vi "precess_SN.vi"() -> ()   [LabVIEW 2010]
panel:
  out "STR":dbl format="%.12g"
  out "DEC 2":dbl caption="DEC 2 [°.xxxxxx]" format="%.6g"
  out "RA 2":dbl caption="RA 2 [h.xxxxxx]" format="%.6g"
  in  "EPOCH2":dbl caption="EPOCH 2" format="%.3g"
  in  "EPOCH1":dbl caption="EPOCH 1" format="%.3g"
  in  "DEC 1":dbl caption="DEC 1 [°.xxxxxx]" format="%.6g"
  in  "RA 1":dbl caption="RA 1 [h.xxxxxx]" format="%.6g"
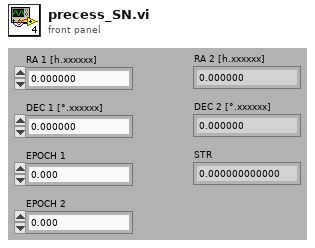
[diagram p1: front panel]
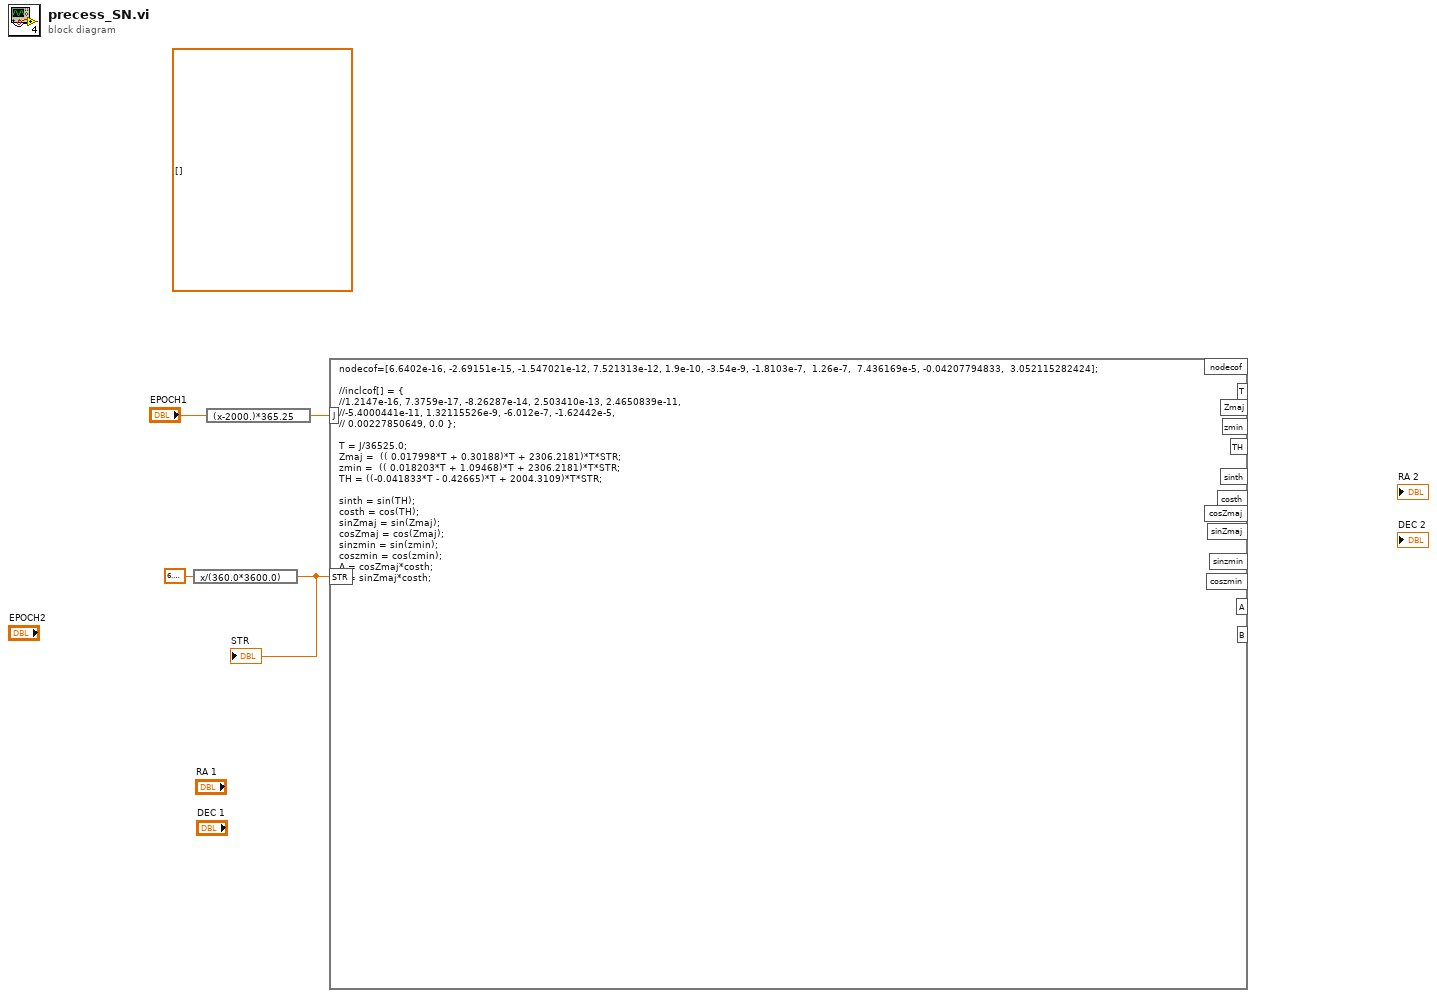
[diagram p0: block diagram]
diagram:
  (unwired) dbl[] []
  n1 = expression code="x/(360.0*3600.0)"(6.283185307179586) -> (w1:dbl)
  "STR" <- w1
  n2 = expression code="(x-2000.)*365.25"("EPOCH1") -> (w3:dbl)
  n3 = formula code="nodecof=[6.6402e-16, -2.69151e-15, -1.547021e-12, 7.521313e-12, 1.9e-10, -3.54e-9, -1.8103e-7,  1.26e-7,  7.436169e-5, -0.04207794833,  3.052115282424];\n\n//inclcof[] = {\n//1.2147e-16, 7.3759e-17, -8.26287e-14, 2.503410e-13, 2.4650839e-11, \n//-5.4000441e-11, 1.32115526e-9, -6.012e-7, -1.62442e-5,\n// 0.00227850649, 0.0 };\n\nT = J/36525.0;\nZmaj =  (( 0.017998*T + 0.30188)*T + 2306.2181)*T*STR;\nzmin =  (( 0.018203*T + 1.09468)*T + 2306.2181)*T*STR;\nTH = ((-0.041833*T - 0.42665)*T + 2004.3109)*T*STR;\n\nsinth = sin(TH);\ncosth = cos(TH);\nsinZmaj = sin(Zmaj);\ncosZmaj = cos(Zmaj);\nsinzmin = sin(zmin);\ncoszmin = cos(zmin);\nA = cosZmaj*costh;\nB = sinZmaj*costh;"("J"=w3, "STR"=w1) -> ()  [unwired: 13 out]
